vi "Set RTDriver VIs File Paths.vi"(8 "error in":errorcluster, 11 "Item Ref in":u64 format="%.0x") -> (0 "error out":errorcluster, 3 "Item Ref out":u64 format="%.0x")   [LabVIEW 2026, in "Template Configuration.lvlib"]
uses:
  Template Configuration.lvlib
  <vilib>/Utility/LVLibp/NI_PackedLibraryUtility.lvlib
  NationalInstruments.VeriStand.SystemStorage
  <vilib>/Utility/error.llb/Trim Whitespace (string).vi
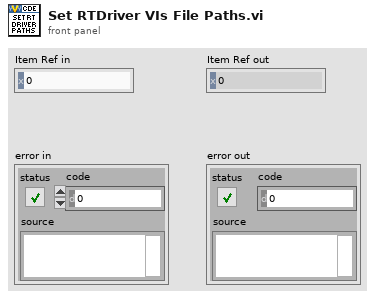
[diagram p1: front panel]
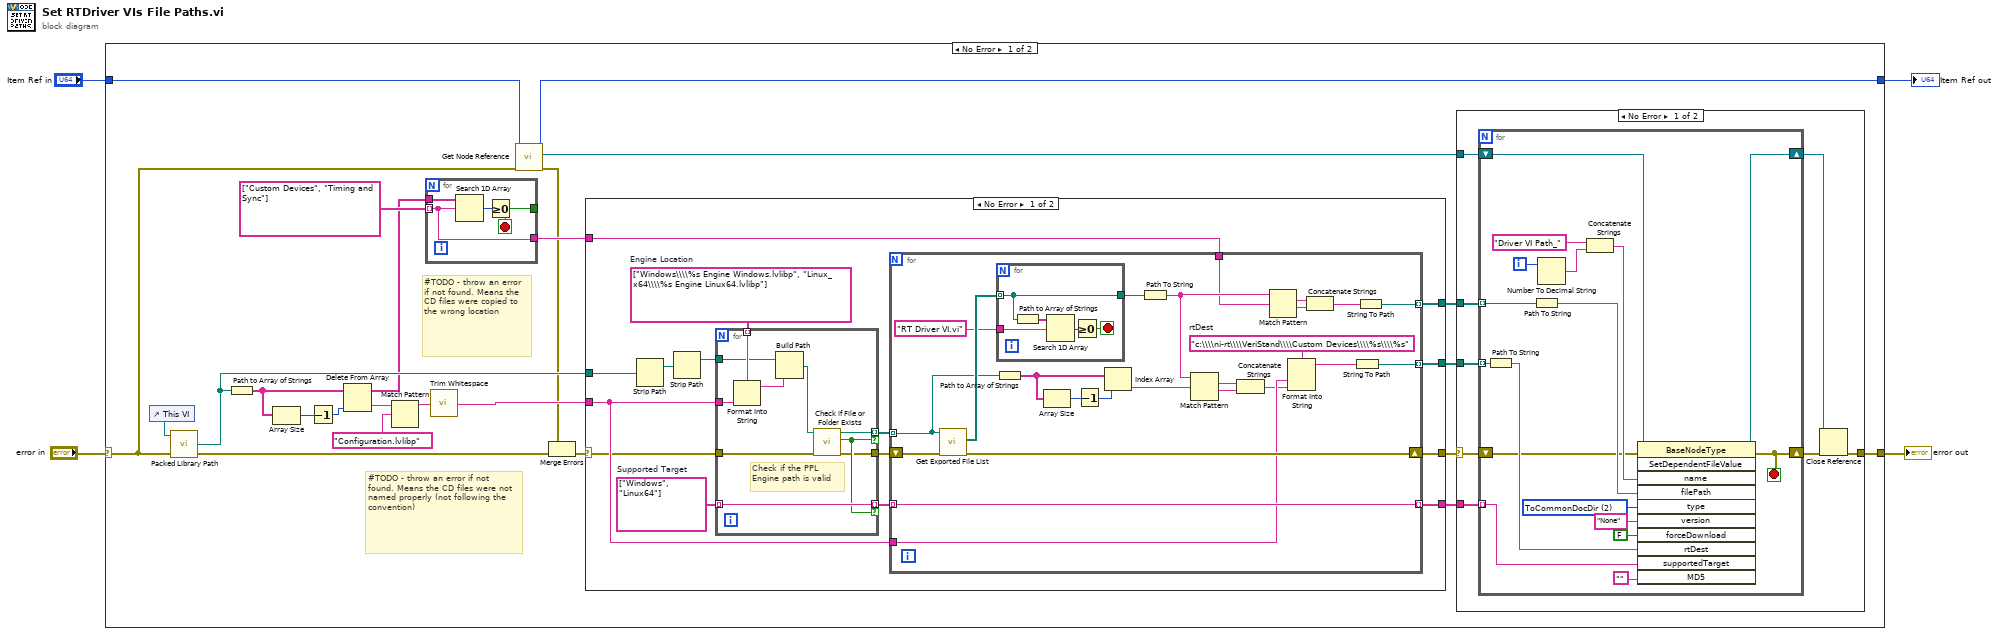
[diagram p0: block diagram]
diagram:
  n1 = case shown="No Error" "error in" {
    selector: "error in" -> [w26 w114]
    tunnel: [w28 w114] -> w4
    tunnel: [w25 w115] -> w3
    tunnel: "Item Ref in" -> [w27 w115]
    frame No Error {
      # "#TODO - throw an error if not found. Means the CD files were not named properly (not following the convention)"
      # "#TODO - throw an error if not found. Means the CD files were copied to the wrong location"
      n2 = control-ref of="This VI"() -> (w24:refnum<vi>)
      n3 = call <vilib>:"Packed Library Path.vi"("error in (no error)"=w26, "vi reference"=w24) -> ("error out"=w7:errorcluster, "packed library path"=w23:path)  [unwired: 1 in, 1 out]
      n4 = Path to Array of Strings(0:w23) -> (2:w22:string[])  [unwired: 1 out]
      n5 = Array Size(array=w22) -> (size(s)=w21:i32)
      n6 = Decrement(x=w21) -> (x-1=w20:i32)
      n7 = Delete From Array(array=w22, index=w20) -> (deleted portion=w19:string, array with subset deleted=w15:string[])  [unwired: 1 in]
      n8 = Match Pattern(string=w19, regular expression="Configuration.lvlibp") -> (before substring=w13:string)  [unwired: 1 in, 3 out]
      n9 = for {
        tunnel: string[] ["Custom Devices", "Timing and Sync"] ("array of strings") -> [w84] mode=indexing
        tunnel: [w86] -> _
        tunnel: w15 -> [w85]
        tunnel: [w84] -> w14
        stop <- w86 stop-if-true
        n10 = Search 1D Array(1D array=w85, element=w84) -> (index of element=w87:i32)  [unwired: 1 in]
        n11 = Greater Or Equal To 0?(x=w87) -> (x >= 0?=w86:bool)
      }
      n12 = call-poly <vilib>:"Trim Whitespace.vi"("string"=w13) -> ("trimmed string"=w17:string)  [unwired: 1 in]
      n13 = call "Get Node Reference.vi"("error in"=w26, "Item Ref in"=w27) -> ("error out"=w6:errorcluster, "Base Node Type"=w5:refnum<k24>, "Item Ref out"=w25:u64)  [unwired: 6 in, 1 out]
      n14 = Merge Errors(w6, w7) -> (w8:errorcluster)
      n15 = case shown="No Error" w8 {
        selector: w8 -> [w32 w83]
        tunnel: w23 -> [w42 _]
        tunnel: [w37 w83] -> w9
        tunnel: w17 -> [w33 _]
        tunnel: w14 -> [w41 _]
        tunnel: [w40 _] -> w12
        tunnel: [w39 _] -> w11
        tunnel: [w38 _] -> w10
        frame No Error {
          w36 = string[] ["Windows\\\\%s Engine Windows.lvlibp", "Linux_x64\\\\%s Engine Linux64.lvlibp"]  # Engine Location
          w34 = string[] ["Windows", "Linux64"]  # Supported Target
          n16 = Strip Path(path=w42) -> (stripped path=w43:path)  [unwired: 1 out]
          n17 = Strip Path(path=w43) -> (stripped path=w35:path)  [unwired: 1 out]
          n18 = for {
            tunnel: w36 -> [w53] mode=indexing
            tunnel: w35 -> [w51]
            tunnel: [w49] -> w29 mode=indexing if=w45
            tunnel: w32 -> [w46]
            tunnel: [w44] -> w31
            tunnel: w34 -> [w48] mode=indexing
            tunnel: [w48] -> w30 mode=indexing if=w45
            tunnel: w33 -> [w47]
            # "Check if the PPL Engine path is valid"
            n19 = Format Into String(format string=w53, w47) -> (resulting string=w52:string)  [unwired: 2 in, 1 out]
            n20 = Build Path(base path=w51, name or relative path=w52) -> (appended path=w50:path)
            n21 = call <vilib>:"Check if File or Folder Exists.vi"("error in (no error)"=w46, "path"=w50) -> ("error out"=w44:errorcluster, "file or folder exists?"=w45:bool, "dup path"=w49:path)  [unwired: 7 in]
          }
          n22 = for {
            shift-right: [w74] -> w37
            shift-left: w31 -> [w75]
            tunnel: w41 -> [w62]
            tunnel: [w61] -> w40 mode=indexing
            tunnel: [w60] -> w39 mode=indexing
            tunnel: [w59] -> w38 mode=indexing
            tunnel: w33 -> [w57]
            tunnel: w30 -> [w59] mode=indexing
            tunnel: w29 -> [w58] mode=indexing
            w54 = "c:\\\\ni-rt\\\\VeriStand\\\\Custom Devices\\\\%s\\\\%s"  # rtDest
            n23 = call <vilib>:"Get Exported File List.vi"("error in (no error)"=w75, "packed library path"=w58) -> ("error out"=w74:errorcluster, "paths"=w77:path[])  [unwired: 7 in, 1 out]
            n24 = Path to Array of Strings(0:w58) -> (2:w65:string[])  [unwired: 1 out]
            n25 = for {
              tunnel: w77 -> [w79] mode=indexing
              tunnel: "RT Driver VI.vi" ("element") -> [w81]
              tunnel: [w79] -> w73
              stop <- w78 stop-if-true
              n26 = Path to Array of Strings(0:w79) -> (2:w82:string[])  [unwired: 1 out]
              n27 = Search 1D Array(1D array=w82, element=w81) -> (index of element=w80:i32)  [unwired: 1 in]
              n28 = Greater Or Equal To 0?(x=w80) -> (x >= 0?=w78:bool)
            }
            n29 = Array Size(array=w65) -> (size(s)=w67:i32)
            n30 = Decrement(x=w67) -> (x-1=w66:i32)
            n31 = Index Array(array=w65, index=w66) -> (element=w64:string)
            n32 = Path To String(path=w73) -> (string=w70:string)
            n33 = Match Pattern(string=w70, regular expression=w64) -> (match substring=w69:string, after substring=w68:string)  [unwired: 1 in, 2 out]
            n34 = Concatenate Strings(w69, w68) -> (w56:string)
            n35 = Match Pattern(string=w70, regular expression=w62) -> (match substring=w72:string, after substring=w71:string)  [unwired: 1 in, 2 out]
            n36 = Format Into String(format string=w54, w57, w56) -> (resulting string=w55:string)  [unwired: 2 in, 1 out]
            n37 = Concatenate Strings(w72, w71) -> (w63:string)
            n38 = String To Path(string=w55) -> (path=w60:path)
            n39 = String To Path(string=w63) -> (path=w61:path)
          }
        }
        frame Error {
        }
      }
      n40 = case shown="No Error" w9 {
        selector: w9 -> [w89 w113]
        tunnel: [w94 w113] -> w28
        tunnel: w12 -> [w93 _]
        tunnel: w11 -> [w92 _]
        tunnel: w10 -> [w91 _]
        tunnel: w5 -> [w90 _]
        frame No Error {
          n41 = for {
            shift-right: [w99] -> w95
            shift-left: w90 -> [w107]
            tunnel: w93 -> [w104] mode=indexing
            tunnel: w92 -> [w103] mode=indexing
            tunnel: w91 -> [w102] mode=indexing
            shift-right: [w96] -> w88
            shift-left: w89 -> [w97]
            i -> [w111]
            stop <- w96 stop-if-true
            w106 = 2 items=["Absolute", "Relative", "ToCommonDocDir", "ToApplicationDataDir"] ("type")
            n42 = Path To String(path=w103) -> (string=w108:string)
            n43 = Path To String(path=w104) -> (string=w109:string)
            n44 = Number To Decimal String(number=w111) -> (decimal integer string=w112:string)  [unwired: 1 in]
            n45 = Concatenate Strings("Driver VI Path_" ("Property name"), w112) -> (w100:string)
            n46 = invoke class="BaseNodeType" method="SetDependentFileValue"(reference=w107, error in=w97, "name"=w100, "filePath"=w109, "type"=w106, "version"="None", "forceDownload"=FALSE, "rtDest"=w108, "supportedTarget"=w102, "MD5"="") -> (reference out=w99:refnum<k24>, error out=w96:errorcluster)  [unwired: 1 in, 9 out]
          }
          n47 = Close Reference(reference=w95, error in (no error)=w88) -> (error out=w94:errorcluster)
        }
        frame Error {
        }
      }
    }
    frame Error {
    }
  }
  "error out" <- w4
  "Item Ref out" <- w3
